vi "File Create HCC.vi"(0 "base path":path, 1 "Station,Data Set ID":string, 2 "Header":string[][](array[string]), 5 "Washer Array":T1[](array[typedef])) -> (4 "appended path":path)   [LabVIEW 2011]
uses:
  HCC Data.ctl
  Washer Status Ctrl.ctl
  <vilib>/Utility/file.llb/Write To Spreadsheet File (string).vi
  Globals HCC.vi
panel:
  out "error out":errorcluster
  in  "error in":errorcluster
  in  "Use Day In Path":bool=TRUE
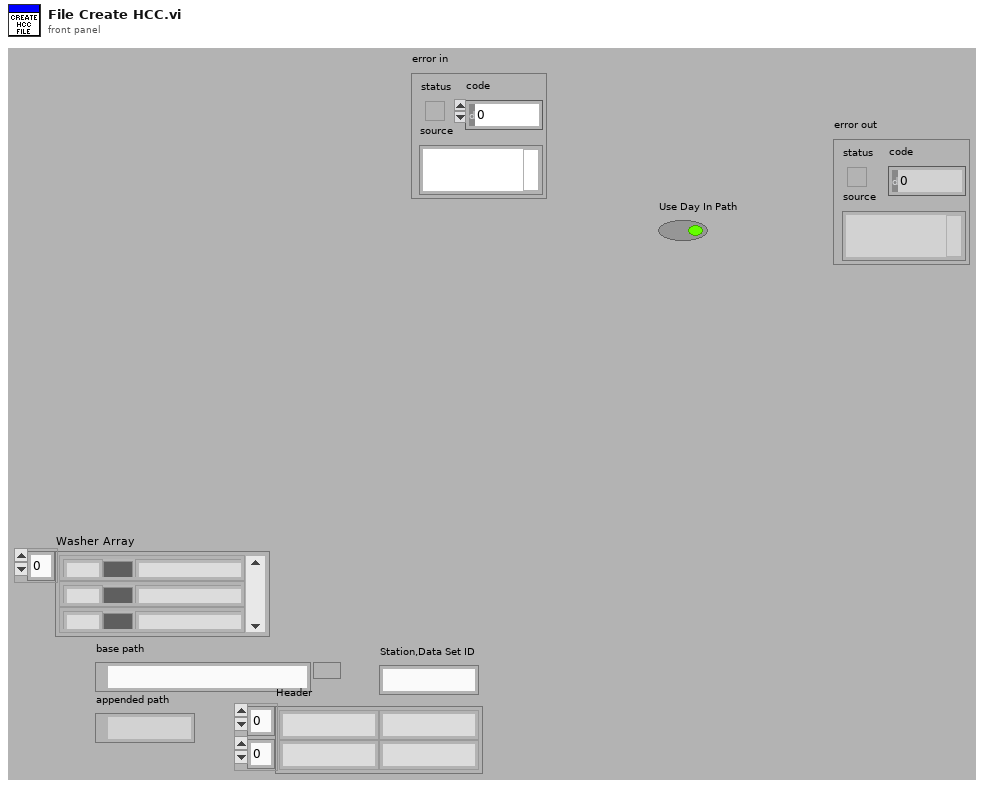
[diagram p1: front panel]
types:
  T1 = typedef "HCC Data.ctl" = cluster{"Station":string, "Color":u32, "Status":T2, "Error Time":string, "Com Err Count":u32, "Debug Log":string}
  T2 = typedef "Washer Status Ctrl.ctl" = enum16{"Running", "Err", "No Com", "No Conf"}
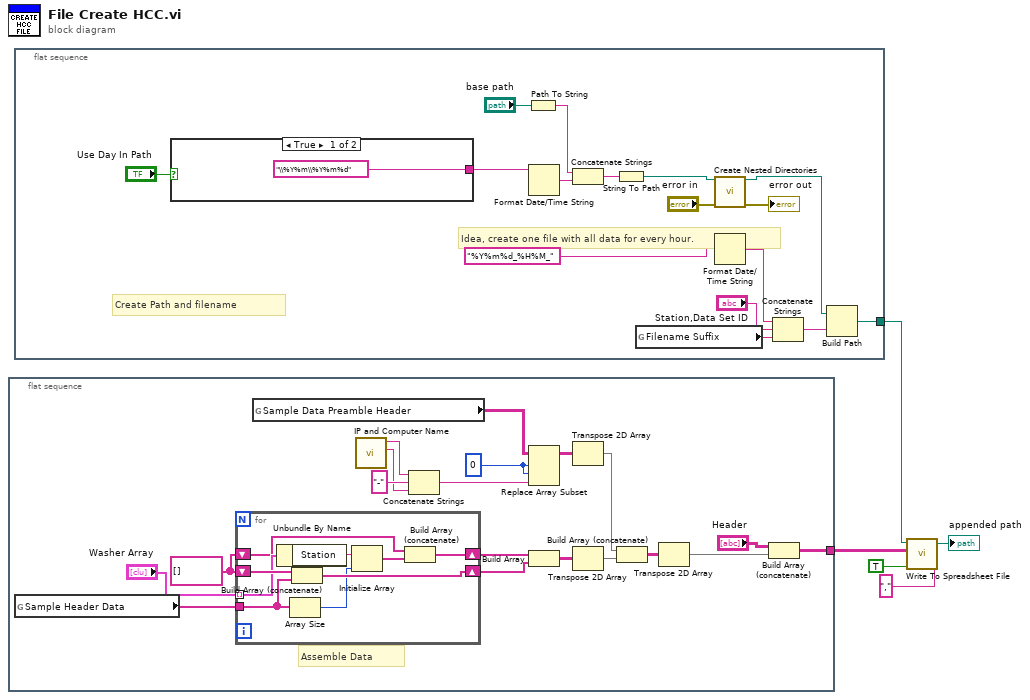
[diagram p0: block diagram]
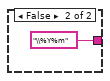
[diagram p2: hidden frame]
diagram:
  n1 = flat-sequence {
    tunnel: [w6] -> w2
    frame #0 {
      w16 = string[] []
      w21 = 0 ("index (row)")
      # "Assemble Data"
      n2 = global read "Globals HCC.vi" "Sample Header Data"() -> (w23:string[])
      n3 = for {
        tunnel: "Washer Array" -> [w32] mode=indexing
        shift-right: [w31] -> w12
        shift-left: w16 -> [w33]
        tunnel: w23 -> [w30]
        shift-right: [w26] -> w11
        shift-left: w16 -> [w25]
        n4 = Unbundle By Name(w32) -> ("Station"=w29:string)
        n5 = Array Size(array=w30) -> (size(s)=w28:i32)
        n6 = Build Array (concatenate)(w33, w30) -> (w31:string[])
        n7 = Initialize Array(w29, w28) -> (w27:string[])
        n8 = Build Array (concatenate)(w25, w27) -> (w26:string[])
      }
      n9 = global read "Globals HCC.vi" "Sample Data Preamble Header"() -> (w22:string[][])
      n10 = call "IP and Computer Name.vi"() -> ("IP Address"=w18:string, "Computer Name"=w20:string)  [unwired: 10 in]
      n11 = Concatenate Strings(w20, "-" ("string"), w18) -> (w17:string)
      n12 = Replace Array Subset(array=w22, new element=w17, index (row)=w21, index (col)=w21) -> (w15:string[][])
      n13 = Build Array(w11, w12) -> (w13:string[][])
      n14 = Transpose 2D Array(2D array=w15) -> (transposed array=w10:string[][])
      n15 = Transpose 2D Array(2D array=w13) -> (transposed array=w14:string[][])
      n16 = Build Array (concatenate)(w10, w14) -> (w9:string[][])
      n17 = Transpose 2D Array(2D array=w9) -> (transposed array=w8:string[][])
      n18 = Build Array (concatenate)("Header", w8) -> (w6:string[][])
    }
  }
  n19 = flat-sequence {
    tunnel: [w35] -> w1
    frame #0 {
      # "Create Path and filename"
      # "Idea, create one file with all data for every hour."
      n20 = case shown="True" "Use Day In Path" {
        tunnel: ["\\%Y%m\\%Y%m%d" ("time format string (%c)") "\\%Y%m" ("time format string (%c)")] -> w37
        frame True {
        }
        frame False {
        }
      }
      n21 = Path To String(path="base path") -> (string=w43:string)
      n22 = Format Date/Time String(time format string (%c)=w37) -> (date/time string=w41:string)  [unwired: 2 out]
      n23 = Concatenate Strings(w43, w41) -> (w42:string)
      n24 = String To Path(string=w42) -> (path=w40:path)
      n25 = global read "Globals HCC.vi" "Filename Suffix"() -> (w48:string)
      n26 = call "Create Nested Directories.vi"("path to create"=w40, "error in"="error in") -> ("created path"=w39:path, "error out"=→"error out":errorcluster)  [unwired: 11 in, 1 out]
      n27 = Format Date/Time String(time format string (%c)="%Y%m%d_%H%M_") -> (date/time string=w47:string)  [unwired: 2 out]
      n28 = Concatenate Strings(w47, "Station,Data Set ID", w48) -> (w34:string)
      n29 = Build Path(base path=w39, name or relative path=w34) -> (appended path=w35:path)
    }
  }
  n30 = call-poly <vilib>:"Write To Spreadsheet File.vi"("delimiter (\\t)"="," ("delimiter (\\t)"), "append to file? (new file:F)"=TRUE, "2D data"=w2, "file path (dialog if empty)"=w1) -> ("new file path (Not A Path if cancelled)"=→"appended path":path)  [unwired: 4 in]
